vi "syringconftest.vi"() -> ()   [LabVIEW 2021]
uses:
  <vilib>/Utility/config.llb/Read Key (Double).vi
  <vilib>/Utility/config.llb/Write Key (Double).vi
  <vilib>/Utility/config.llb/NI_LVConfig.lvlib
  <vilib>/Utility/xml.llb/Write to XML File(string).vi
  <vilib>/Utility/xml.llb/Read From XML File(array).vi
panel:
  in  "configuration file in":path
  out "All Found":bool
  out "Read 2":T1(array[cluster])
  in  "Write":T1(array[cluster])
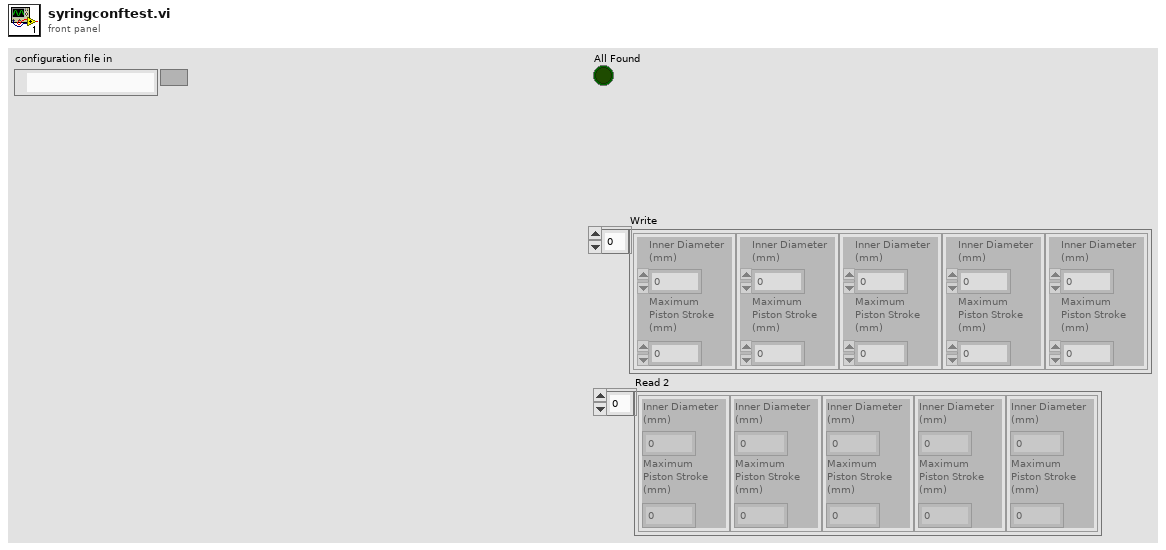
[diagram p1: front panel]
types:
  T1 = cluster{"Inner Diameter \n(mm)":dbl, "Maximum \nPiston Stroke \n(mm)":dbl}[]
  T2 = typedef "NI_LVConfig.lvlib/Config Data RefNum.ctl" = refnum<k1>
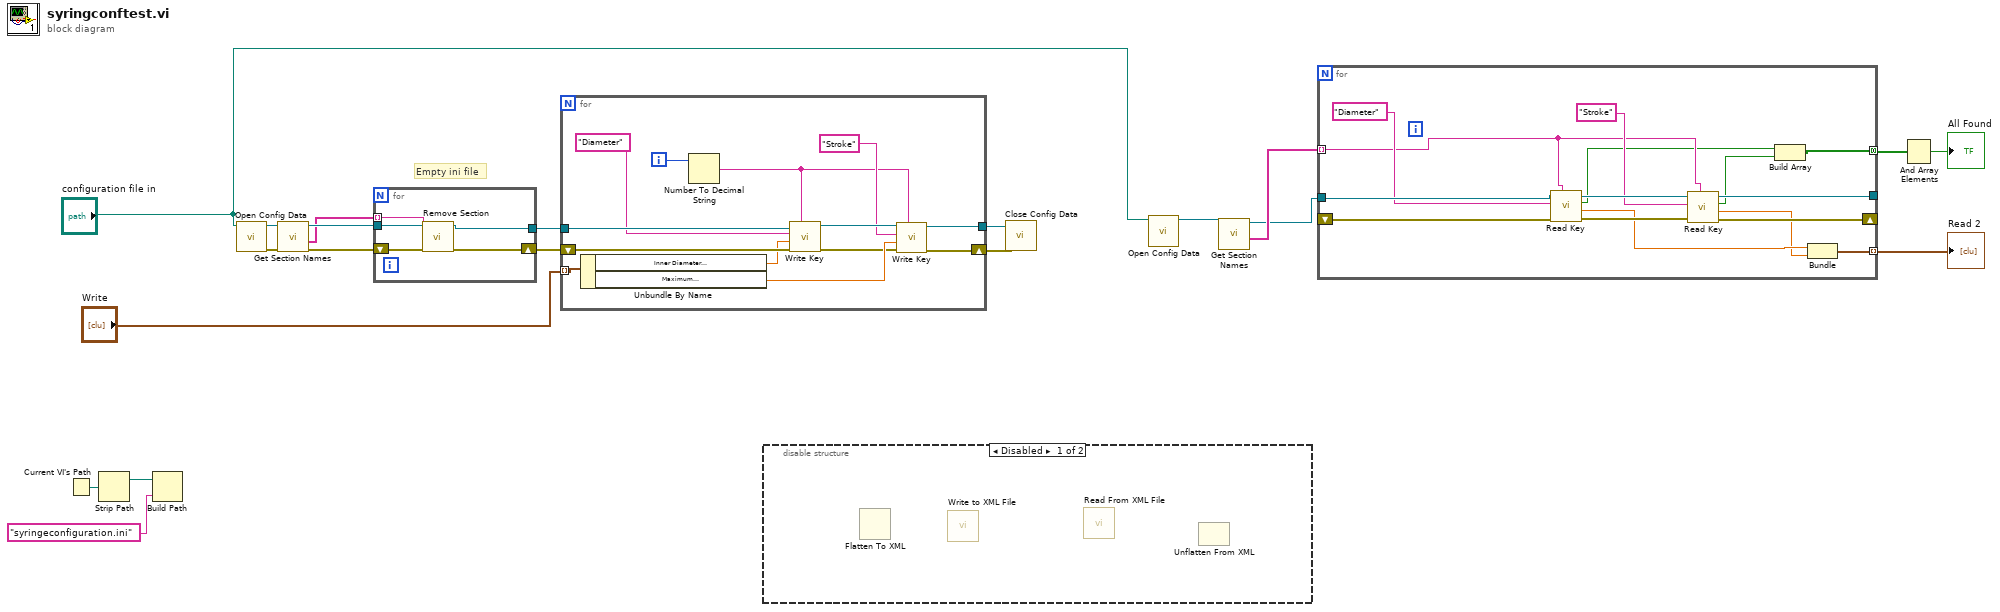
[diagram p0: block diagram]
diagram:
  # "Empty ini file"
  n1 = Current VI's Path() -> (path=w18:path)
  n2 = Strip Path(path=w18) -> (stripped path=w19:path)  [unwired: 1 out]
  n3 = Build Path(base path=w19, name or relative path="syringeconfiguration.ini") -> ()  [unwired: 1 out]
  n4 = call <vilib>:"Open Config Data.vi"("configuration file path"="configuration file in") -> ("error out"=w10:errorcluster, "refnum"=w17:T2)  [unwired: 8 in, 1 out]
  n5 = call <vilib>:"Get Section Names.vi"("error in (no error)"=w10, "refnum"=w17) -> ("error out"=w14:errorcluster, "section names"=w15:string[], "refnum out"=w16:T2)  [unwired: 7 in]
  n6 = for {
    tunnel: w16 -> [w25]
    tunnel: w15 -> [w24] mode=indexing
    tunnel: [w21] -> w12
    shift-right: [w22] -> w13
    shift-left: w14 -> [w23]
    n7 = call <vilib>:"Remove Section.vi"("section"=w24, "error in (no error)"=w23, "refnum"=w25) -> ("error out"=w22:errorcluster, "refnum out"=w21:T2)  [unwired: 6 in, 1 out]
  }
  n8 = for {
    tunnel: w12 -> [w37]
    tunnel: "Write" -> [w33] mode=indexing
    tunnel: [w28] -> w9
    shift-right: [w27] -> w8
    shift-left: w13 -> [w38]
    i -> [w30]
    n9 = Unbundle By Name(w33) -> ("Inner Diameter \n(mm)"=w32:dbl, "Maximum \nPiston Stroke \n(mm)"=w31:dbl)
    n10 = Number To Decimal String(number=w30) -> (decimal integer string=w29:string)  [unwired: 1 in]
    n11 = call-poly <vilib>:"Write Key.vi"("section"=w29, "error in (no error)"=w38, "value"=w32, "key"="Diameter", "refnum"=w37) -> ("error out"=w26:errorcluster, "refnum out"=w36:T2)  [unwired: 4 in, 1 out]
    n12 = call-poly <vilib>:"Write Key.vi"("section"=w29, "error in (no error)"=w26, "value"=w31, "key"="Stroke", "refnum"=w36) -> ("error out"=w27:errorcluster, "refnum out"=w28:T2)  [unwired: 4 in, 1 out]
  }
  n13 = disable-structure shown="Disabled" {
    frame Disabled {
      n14 = Flatten To XML() -> ()  [unwired: 1 in, 1 out]
      n15 = call-poly <vilib>:"Write to XML File.vi"() -> ()  [unwired: 9 in, 3 out]
      n16 = call-poly <vilib>:"Read From XML File.vi"() -> ()  [unwired: 9 in, 3 out]
      n17 = Unflatten From XML() -> ()  [unwired: 3 in, 2 out]
    }
    frame Enabled {
    }
  }
  n18 = call <vilib>:"Close Config Data.vi"("error in (no error)"=w8, "refnum"=w9) -> ()  [unwired: 8 in, 2 out]
  n19 = call <vilib>:"Open Config Data.vi"("configuration file path"="configuration file in") -> ("refnum"=w7:T2)  [unwired: 8 in, 2 out]
  n20 = call <vilib>:"Get Section Names.vi"("refnum"=w7) -> ("section names"=w6:string[], "refnum out"=w5:T2)  [unwired: 8 in, 1 out]
  n21 = for {
    tunnel: w5 -> [w53]
    tunnel: [w51] -> _
    shift-right: [w50] -> _
    shift-left: _ -> [w48]
    tunnel: w6 -> [w42] mode=indexing
    tunnel: [w43] -> w4 mode=indexing
    tunnel: [w39] -> w3 mode=concatenating
    n22 = call-poly <vilib>:"Read Key.vi"("section"=w42, "error in (no error)"=w48, "key"="Diameter", "refnum"=w53) -> ("error out"=w49:errorcluster, "value"=w45:dbl, "found?"=w41:bool, "refnum out"=w52:T2)  [unwired: 4 in]
    n23 = call-poly <vilib>:"Read Key.vi"("section"=w42, "error in (no error)"=w49, "key"="Stroke", "refnum"=w52) -> ("error out"=w50:errorcluster, "value"=w44:dbl, "found?"=w40:bool, "refnum out"=w51:T2)  [unwired: 4 in]
    n24 = Build Array(w41, w40) -> (w39:bool[])
    n25 = Bundle("value"=w45, "value"=w44) -> (w43:cluster{"value":dbl, "value":dbl})  [unwired: 1 in]
  }
  "Read 2" <- w4
  n26 = And Array Elements(Boolean array=w3) -> (logical AND=→"All Found":bool)
